vi "excelSavesubVI.vi"   [LabVIEW 2012]
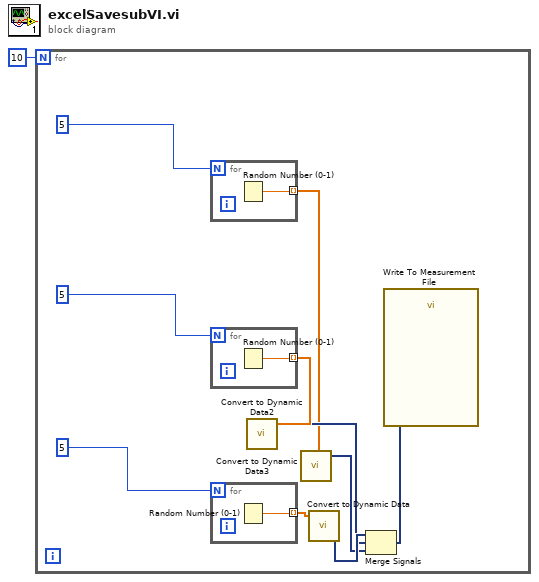
[diagram p0: block diagram]
diagram:
  n1 = for {
    N: 10 -> [_]
    n2 = for {
      N: 5 -> [_]
      tunnel: [w14] -> w3 mode=indexing
      n3 = Random Number (0-1)() -> (number: 0 to 1=w14:dbl)
    }
    n4 = for {
      N: 5 -> [_]
      tunnel: [w13] -> w5 mode=indexing
      n5 = Random Number (0-1)() -> (number: 0 to 1=w13:dbl)
    }
    n6 = for {
      N: 5 -> [_]
      tunnel: [w12] -> w8 mode=indexing
      n7 = Random Number (0-1)() -> (number: 0 to 1=w12:dbl)
    }
    n8 = call "Convert to Dynamic Data2"("Array"=w5) -> ("Dynamic Data Type"=w4:dynamicdata)  [unwired: 3 in]
    n9 = call "Convert to Dynamic Data3"("Array"=w3) -> ("Dynamic Data Type"=w2:dynamicdata)  [unwired: 3 in]
    n10 = call "Convert to Dynamic Data"("Array"=w8) -> ("Dynamic Data Type"=w7:dynamicdata)  [unwired: 3 in]
    n11 = Merge Signals(w7, w4, w2) -> (w6:dynamicdata)
    n12 = call "Write To Measurement File"("Signals"=w6) -> ()  [unwired: 16 in, 3 out]
  }
